vi "Do.vi"(8 "error in (no error)":errorcluster, 10 "Actor in":refnum<class "Actor.lvclass">, 11 "DNL_Message Template":refnum<class "New Image Msg.lvclass">) -> (0 "error out":errorcluster, 2 "Actor out":refnum<class "Actor.lvclass">)   [LabVIEW 2014, in "Storage.lvlib" / "New Image Msg.lvclass"]
doc: "This VI delivers the message to the actor by calling the appropriate method(s) on the actor."
uses:
  New Image Msg.lvclass
  <vilib>/ActorFramework/Actor/Actor.lvclass
  Storage/Storage.lvclass
  Camera Actors/Camera Actor/Camera Actor Messages/New Image Msg/New Image Msg.lvclass/New Image Msg.ctl
  Camera Actors/Camera Actor/Camera Actor Messages/New Image Msg/New Image Msg.lvclass
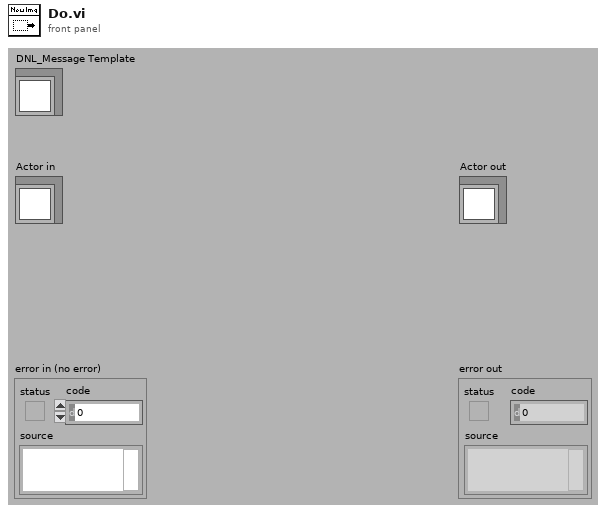
[diagram p1: front panel]
types:
  T1 = typedef "IMAQ Image.ctl" = refnum<image>
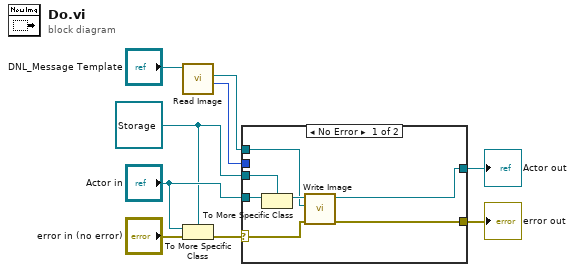
[diagram p0: block diagram]
diagram:
  w1 = refnum<class "Storage.lvclass"> refnum ("Storage.lvlib:Storage.lvclass")
  n1 = call "Read Image.vi"("New Image Msg in"="DNL_Message Template") -> ("Buffer Number"=w2:u32, "Image"=w3:T1)  [unwired: 7 in, 2 out]
  n2 = To More Specific Class(target class=w1, reference="Actor in", error in="error in (no error)") -> (error out=w8:errorcluster)  [unwired: 1 out]
  n3 = case shown="No Error" w8 {
    selector: w8 -> [w14 w18]
    tunnel: [w16 w18] -> w7
    tunnel: [w15 w17] -> w6
    tunnel: "Actor in" -> [w13 w17]
    tunnel: w1 -> [w12 _]
    tunnel: w3 -> [w10 _]
    tunnel: w2 -> [_ _]
    frame No Error {
      n4 = To More Specific Class(target class=w12, reference=w13) -> (specific class reference=w11:refnum<class "Storage.lvclass">)  [unwired: 1 in, 1 out]
      n5 = call-dynamic "Write Image.vi"("error in (no error)"=w14, "Image"=w10, "Storage in"=w11) -> ("error out"=w16:errorcluster, "Storage out"=w15:refnum<class "Storage.lvclass">)  [unwired: 7 in]
    }
    frame Error {
      # "If type check fails, pass the original object out again."
    }
  }
  "error out" <- w7
  "Actor out" <- w6
